vi "UpdateLastLoadedFile.vi"(0 "LoadOrSave":enum16{"Load", "Save"}(ring), 9 "GUIName":string, 11 "FileNameIn":string, 12 "error IO":errorcluster) -> ()   [LabVIEW 2014, in "Panels.lvlib"]
uses:
  Panels.lvlib
  CS_Core/CSSystem/CoreDefs/CoreDefs.call_type.ctl
  CS_Core/BaseProcess/BaseProcess.descriptor string definition.ctl
  CS_Core/CSSystem/CoreDefs/CoreDefs.rawDataType.ctl
  CS_Core/CSSystem/CoreLib/CoreLib.string 2 byte array.vi
  CS_Core/CSSystem/CoreLib/CoreLib.short 2 byte array.vi
  Instance           2 28Saved   UpdateLastLoadedFile .vi
  CS_Core/CSSystem/CoreLib/CoreLib.lvlib
  CS_Core/BaseProcess/BaseProcess.lvlib
panel:
  in  "call cluster in":T1={"Object"="", "Selector"="", "CallType"=enum."synchronous", "Async Object"="", "Async Selector"="", "Data Descriptor"="", "Data"=[], "Error #"=0, "Expire"=0}
  out "error out":errorcluster
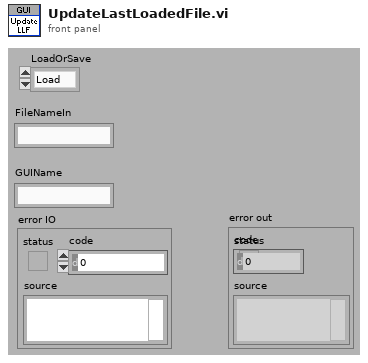
[diagram p1: front panel]
types:
  T1 = typedef "CoreDefs.call_type.ctl" = cluster{"Object":string, "Selector":string, "CallType":enum16{"simple", "synchronous", "asynchronous"}, "Async Object":string, "Async Selector":string, "Data Descriptor":T2, "Data":T3, "Error #":i32, "Expire":u32}
  T2 = typedef "BaseProcess.lvlib/BaseProcess.descriptor string definition.ctl" = string
  T3 = typedef "CoreDefs.rawDataType.ctl" = i8[]
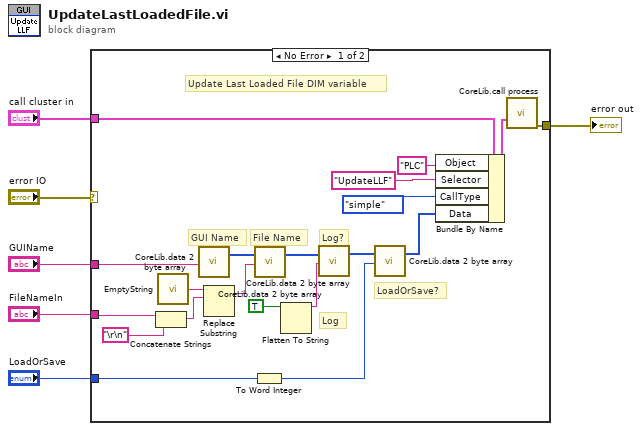
[diagram p0: block diagram]
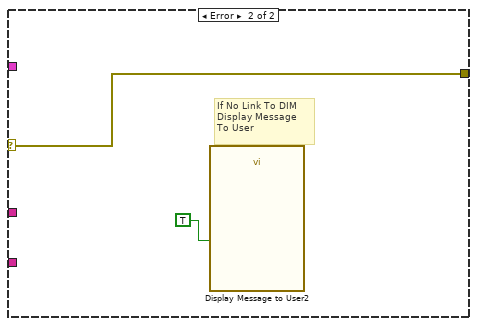
[diagram p2: hidden frame]
diagram:
  n1 = case shown="No Error" "error IO" {
    selector: "error IO" -> [_ w28]
    tunnel: "FileNameIn" -> [w15 _]
    tunnel: "GUIName" -> [w26 _]
    tunnel: [w25 w28] -> w4
    tunnel: "call cluster in" -> [w24 _]
    tunnel: "LoadOrSave" -> [w8 _]
    frame No Error {
      # "LoadOrSave?"
      # "Log?"
      # "File Name"
      # "GUI Name"
      # "Log"
      # "Update Last Loaded File DIM variable"
      n2 = Concatenate Strings(w15, "\r\n") -> (w17:string)
      n3 = call "EmptyString.vi"() -> ("String"=w18:string)
      n4 = call-poly "CoreLib.data 2 byte array.vi"("string"=w26) -> ("byteArray out"=w19:T3)  [unwired: 18 in]
      n5 = Replace Substring(4:w17, 5:w18) -> (1:w14:string)  [unwired: 2 in, 1 out]
      n6 = To Word Integer(number=w8) -> (16bit integer=w7:i16)
      n7 = call-poly "CoreLib.data 2 byte array.vi"("byteArray"=w19, "string"=w14) -> ("byteArray out"=w12:T3)  [unwired: 17 in]
      n8 = Flatten To String(anything=TRUE) -> (data string=w11:string)  [unwired: 3 in, 2 out]
      n9 = call-poly "CoreLib.data 2 byte array.vi"("byteArray"=w12, "string"=w11) -> ("byteArray out"=w10:T3)  [unwired: 17 in]
      n10 = call-poly "CoreLib.data 2 byte array.vi"("byteArray"=w10, "i16"=w7) -> ("byteArray out"=w9:T3)  [unwired: 17 in]
      n11 = Bundle By Name(cluster=w24, "Object"="PLC", "Selector"="UpdateLLF" ("serviceName"), "CallType"=enum16{"simple", "synchronous", "asynchronous"}."simple", "Data"=w9) -> (w23:T1)
      n12 = call "CoreLib.call process.vi"("call cluster in"=w23) -> ("error out"=w25:errorcluster)  [unwired: 13 in, 1 out]
    }
    frame Error {
      # "If No Link To DIM \nDisplay Message\nTo User"
      n13 = call "Display Message to User2"("Enable"=TRUE) -> ()  [unwired: 9 in, 2 out]
    }
  }
  "error out" <- w4
